vi "Dispose Report.vi"(0 "report in":refnum<class "NI_Standard Report.lvclass">, 5 "wait until printing completed? (T)":bool=TRUE, 9 "save changes? (F)":bool, 11 "error in (no error)":errorcluster, 12 "close report? (T)":bool=TRUE) -> (15 "error out":errorcluster)   [LabVIEW 2015, in "NI_Standard Report.lvclass"]
doc: "Closes the report and releases its interface, which saves memory."
uses:
  <vilib>/Utility/NIReport.llb/Standard Report/NI_Standard Report.lvclass
  <vilib>/Utility/NIReport.llb/Standard Report/NI_Standard Report.lvclass/NI_Standard Report.ctl
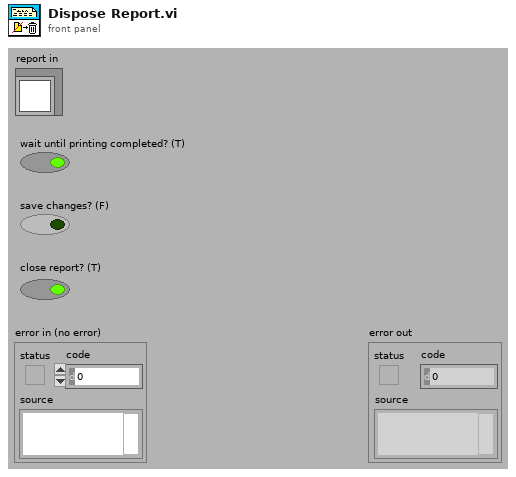
[diagram p1: front panel]
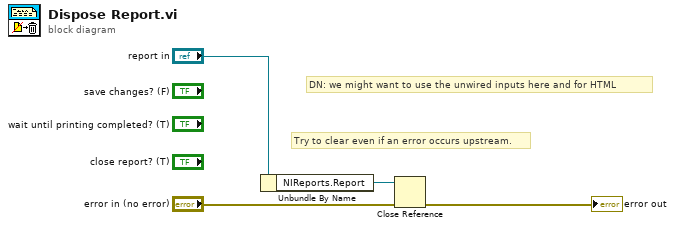
[diagram p0: block diagram]
diagram:
  # "DN: we might want to use the unwired inputs here and for HTML"
  # "Try to clear even if an error occurs upstream."
  n1 = Unbundle By Name("report in") -> ("NIReports.Report"=w1:refnum<k7>)
  n2 = Close Reference(reference=w1, error in (no error)="error in (no error)") -> (error out=→"error out":errorcluster)
